vi "C-V 曲线测试.vi"() -> ()   [LabVIEW 2011]
panel:
  out "XY图":cluster{dbl[], dbl[]}[](graph)
  in  "测试时间（h）":dbl=0.5
  in  "低温循环测试":bool
  in  "延时（ms）":u32=100
  in  "步进电压(V)":dbl=2.0
  in  "最小电压(V)":dbl
  in  "最大电压(V)":dbl=30.0
  out "error out":errorcluster caption="错误输出"
  in  "Completion Task":u16(ring) caption="完成任务" items=["保持Excel打开", "关闭电子表格"]
  out "错误输出 2":errorcluster caption="错误输出"
  out "错误输出":errorcluster
  in  "Filename":string="TEST"
  in  "第n次记录":dbl
  in  "UNIT":string(combo)="1000000000000"
  in  "错误输入（无错误）":errorcluster
  in  "VISA资源名称":refnum<visa-resource-name>="GPIB0::1::INSTR"
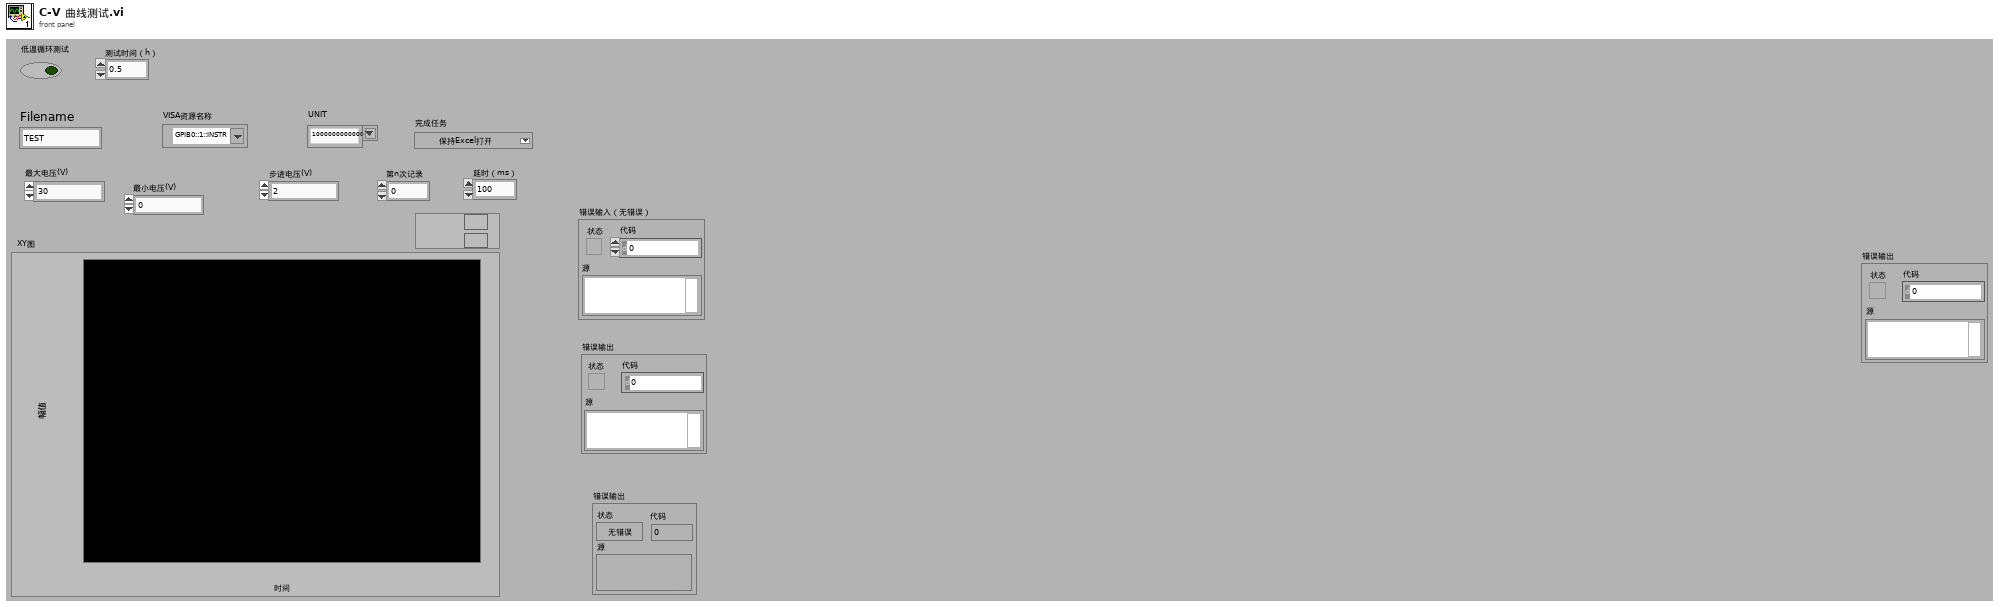
[diagram p1: front panel]
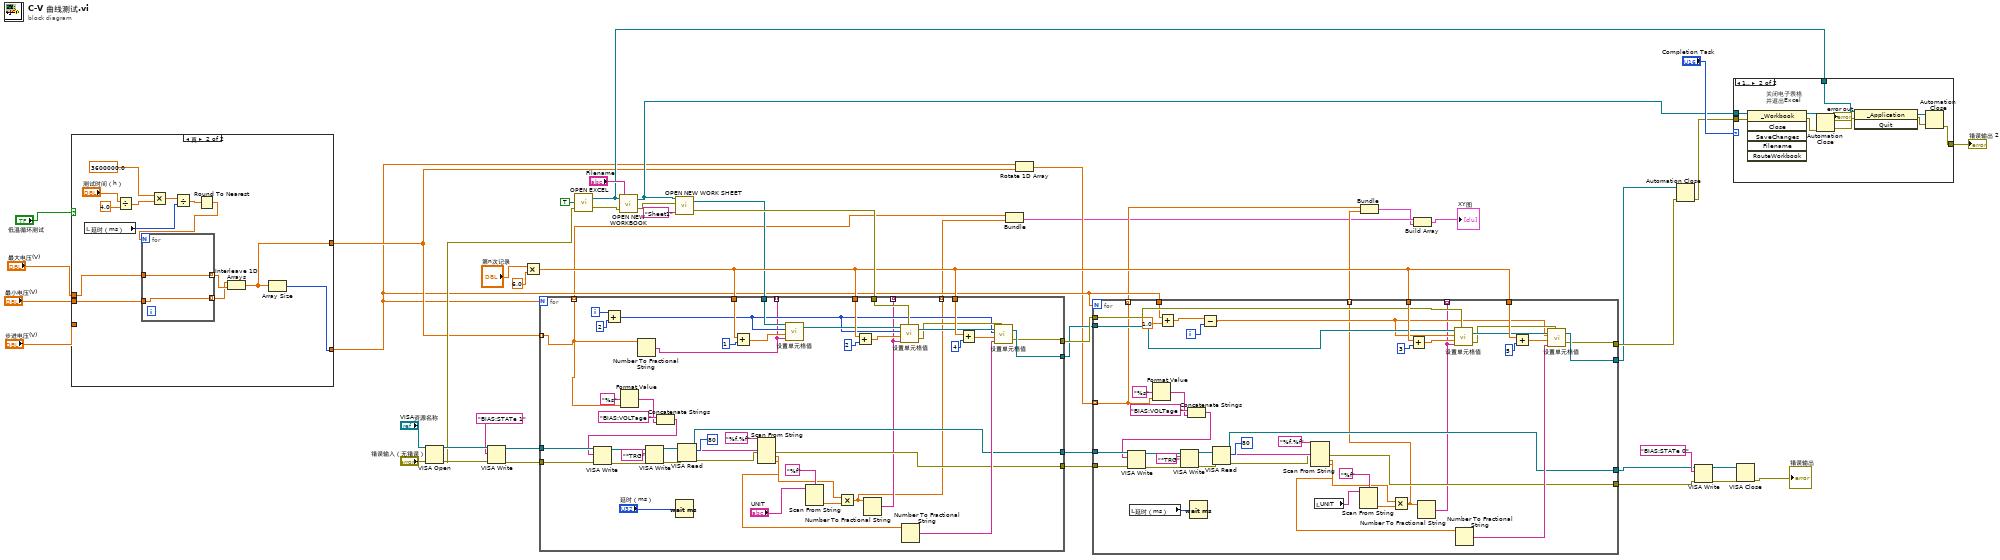
[diagram p0: block diagram]
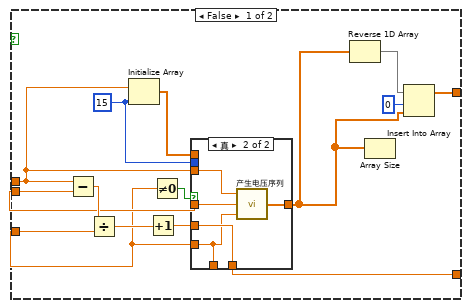
[diagram p2: hidden frame]
diagram:
  n1 = case shown="真" "低温循环测试" {
    tunnel: "最小电压(V)" -> [w53 w83]
    tunnel: "步进电压(V)" -> [w52 _]
    tunnel: "最大电压(V)" -> [w51 w84]
    tunnel: [w50 w74] -> w11
    tunnel: [w49 w73] -> w10
    frame False {
      w56 = 15 ("维数大小")
      n2 = Subtract(x=w51, y=w53) -> (x-y=w62:dbl)
      n3 = Divide(x=w62, y=w52) -> (x/y=w61:dbl)
      n4 = Initialize Array(w51, w56) -> (w57:dbl[])
      n5 = Increment(x=w61) -> (x+1=w58:dbl)
      n6 = Not Equal To 0?(x=w52) -> (x != 0?=w55:bool)
      n7 = case shown="真" w55 {
        tunnel: w53 -> [_ w70]
        tunnel: w51 -> [_ w69]
        tunnel: w52 -> [w63 w66]
        tunnel: [w65 w68] -> w54
        tunnel: w58 -> [_ w67]
        tunnel: [w64 w67] -> w49
        tunnel: w57 -> [w65 _]
        tunnel: w56 -> [w64 _]
        tunnel: [w63 w66] -> _
        frame False {
        }
        frame True {
          n8 = call "产生电压序列.vi"("Delt"=w66, "Min"=w70, "Max"=w69) -> ("Array"=w68:dbl[])
        }
      }
      n9 = Reverse 1D Array(array=w54) -> (reversed array=w59:dbl[])
      n10 = Array Size(array=w54) -> ()  [unwired: 1 out]
      n11 = Insert Into Array(array=w59, index=0 ("索引"), new element=w54) -> (w50:dbl[])
    }
    frame True {
      n12 = local read "延时（ms）"() -> (w77:u32)
      n13 = Divide(x="测试时间（h）", y=4.0) -> (x/y=w80:dbl)
      n14 = Multiply(x=3600000.0, y=w80) -> (x*y=w78:dbl)
      n15 = Divide(x=w78, y=w77) -> (x/y=w76:dbl)
      n16 = Round To Nearest(number=w76) -> (nearest integer value=w75:dbl)
      n17 = for {
        N: w75 -> [_]
        tunnel: w83 -> [w85]
        tunnel: w84 -> [w86]
        tunnel: [w86] -> w72 mode=indexing
        tunnel: [w85] -> w71 mode=indexing
      }
      n18 = Interleave 1D Arrays(w71, w72) -> (w74:dbl[])
      n19 = Array Size(array=w74) -> (size(s)=w73:i32)
    }
  }
  n20 = VISA Open(error in (no error)="错误输入（无错误）", VISA resource name="VISA资源名称") -> (VISA resource name=w47:refnum<visa-resource-name>, error out=w39:errorcluster)  [unwired: 3 in]
  n21 = VISA Write(VISA resource name=w47, write buffer="BIAS:STATe 1" ("写入缓冲区"), error in (no error)=w39) -> (VISA resource name out=w46:refnum<visa-resource-name>, error out=w45:errorcluster)  [unwired: 1 out]
  n22 = Multiply(x="第n次记录", y=6.0) -> (x*y=w22:dbl)
  n23 = call "OPEN EXCEL.vi"("错误输入（无错误）"=w39, "Visible"=TRUE) -> ("错误输出"=w38:errorcluster, "引用输出"=w30:refnum<k7>)  [unwired: 1 in]
  n24 = call "OPEN NEW WORKBOOK.vi"("错误输入（无错误）"=w38, "Filename"="Filename", "Excel._Application"=w30) -> ("错误输出"=w27:errorcluster, "Excel._Application 2"=w28:refnum<k7>)
  n25 = call "OPEN NEW WORK SHEET.vi"("Sheet?"="Sheet1", "错误输入（无错误）"=w27, "Excel._Workbook"=w28) -> ("错误输出"=w25:errorcluster, "Excel._Worksheet"=w21:refnum<k7>)  [unwired: 1 in]
  n26 = for {
    N: w10 -> [_]
    tunnel: w46 -> [w133]
    tunnel: w45 -> [w132]
    tunnel: w22 -> [w114]
    tunnel: w22 -> [w110]
    tunnel: [w100] -> w23
    tunnel: [w103] -> w16
    tunnel: [w102] -> w24
    tunnel: [w101] -> w17
    tunnel: w21 -> [w98]
    tunnel: w25 -> [w99]
    tunnel: w22 -> [w94]
    tunnel: w11 -> [w87] mode=indexing
    tunnel: [w90] -> _ mode=indexing
    tunnel: [w89] -> _ mode=indexing
    tunnel: [w88] -> w6 mode=indexing
    tunnel: [w87] -> w7 mode=indexing
    i -> [w108]
    n27 = Add(x=w108, y=2) -> (x+y=w93:i32)
    n28 = Format Value(format string="%s" ("格式字符串"), value (0)=w87) -> (output string=w124:string)  [unwired: 1 in]
    n29 = Number To Fractional String(number=w87) -> (F-format string=w90:string)  [unwired: 3 in]
    n30 = Concatenate Strings("BIAS:VOLTage " ("字符串"), w124) -> (w123:string)
    n31 = VISA Write(VISA resource name=w133, write buffer=w123, error in (no error)=w132) -> (VISA resource name out=w131:refnum<visa-resource-name>, error out=w130:errorcluster)  [unwired: 1 out]
    n32 = VISA Write(VISA resource name=w131, write buffer="*TRG" ("写入缓冲区"), error in (no error)=w130) -> (VISA resource name out=w129:refnum<visa-resource-name>, error out=w128:errorcluster)  [unwired: 1 out]
    n33 = Wait (ms)(milliseconds to wait="延时（ms）") -> ()  [unwired: 1 out]
    n34 = VISA Read(VISA resource name=w129, byte count=u32 80 ("字节总数"), error in (no error)=w128) -> (VISA resource name out=w102:refnum<visa-resource-name>, read buffer=w121:string, error out=w119:errorcluster)  [unwired: 1 out]
    n35 = Add(x=w94, y=1) -> (x+y=w95:dbl)
    n36 = Scan From String(format string="%f,%f" ("格式字符串"), input string=w121, error in=w119) -> (error out=w100:errorcluster, output 1=w116:dbl, output 2=w105:dbl)  [unwired: 3 in, 2 out]
    n37 = call "设置单元格值.vi"("Excel._Worksheet 2"=w98, "Row"=w93, "Col"=w95, "Value"=w90) -> ("Excel._Worksheet"=w97:refnum<k7>)  [unwired: 1 in, 1 out]
    n38 = Scan From String(format string="%f" ("格式字符串"), input string="UNIT") -> (output 1=w117:dbl)  [unwired: 3 in, 3 out]
    n39 = Multiply(x=w116, y=w117) -> (x*y=w88:dbl)
    n40 = Add(x=w114, y=2) -> (x+y=w113:dbl)
    n41 = Number To Fractional String(number=w88) -> (F-format string=w89:string)  [unwired: 3 in]
    n42 = call "设置单元格值.vi"("Excel._Worksheet 2"=w97, "Row"=w93, "Col"=w113, "Value"=w89, "error in (no error)"=w99) -> ("Excel._Worksheet"=w107:refnum<k7>, "error out"=w106:errorcluster)
    n43 = Number To Fractional String(number=w105) -> (F-format string=w104:string)  [unwired: 3 in]
    n44 = Add(x=w110, y=4) -> (x+y=w112:dbl)
    n45 = call "设置单元格值.vi"("Excel._Worksheet 2"=w107, "Row"=w93, "Col"=w112, "Value"=w104, "error in (no error)"=w106) -> ("Excel._Worksheet"=w103:refnum<k7>, "error out"=w101:errorcluster)
  }
  n46 = Bundle(w7, w6) -> (w3:cluster{dbl[], dbl[]})  [unwired: 1 in]
  n47 = Rotate 1D Array(1:w11, 2:w10) -> (0:w9:dbl[])
  n48 = for {
    N: w10 -> [_]
    tunnel: w24 -> [w177]
    tunnel: w23 -> [w176]
    tunnel: w22 -> [w158]
    tunnel: w22 -> [w154]
    tunnel: [w146] -> w19
    tunnel: [w149] -> w15
    tunnel: [w148] -> w20
    tunnel: [w147] -> w18
    tunnel: w17 -> [w145]
    tunnel: w16 -> [w144]
    tunnel: w10 -> [w140]
    tunnel: [w136] -> _ mode=indexing
    tunnel: w9 -> [w135] mode=indexing
    tunnel: [w135] -> w5 mode=indexing
    tunnel: [w134] -> w4 mode=indexing
    i -> [w141]
    n49 = local read "延时（ms）"() -> (w137:u32)
    n50 = Format Value(format string="%s" ("格式字符串"), value (0)=w135) -> (output string=w168:string)  [unwired: 1 in]
    n51 = Add(x=w140, y=1.0) -> (x+y=w142:dbl)
    n52 = Concatenate Strings("BIAS:VOLTage " ("字符串"), w168) -> (w167:string)
    n53 = VISA Write(VISA resource name=w177, write buffer=w167, error in (no error)=w176) -> (VISA resource name out=w175:refnum<visa-resource-name>, error out=w174:errorcluster)  [unwired: 1 out]
    n54 = VISA Write(VISA resource name=w175, write buffer="*TRG" ("写入缓冲区"), error in (no error)=w174) -> (VISA resource name out=w173:refnum<visa-resource-name>, error out=w172:errorcluster)  [unwired: 1 out]
    n55 = Wait (ms)(milliseconds to wait=w137) -> ()  [unwired: 1 out]
    n56 = Subtract(x=w142, y=w141) -> (x-y=w138:dbl)
    n57 = VISA Read(VISA resource name=w173, byte count=u32 80 ("字节总数"), error in (no error)=w172) -> (VISA resource name out=w148:refnum<visa-resource-name>, read buffer=w165:string, error out=w163:errorcluster)  [unwired: 1 out]
    n58 = Scan From String(format string="%f,%f" ("格式字符串"), input string=w165, error in=w163) -> (error out=w146:errorcluster, output 1=w160:dbl, output 2=w151:dbl)  [unwired: 3 in, 2 out]
    n59 = local read "UNIT"() -> (w143:string)
    n60 = Scan From String(format string="%f" ("格式字符串"), input string=w143) -> (output 1=w161:dbl)  [unwired: 3 in, 3 out]
    n61 = Multiply(x=w160, y=w161) -> (x*y=w134:dbl)
    n62 = Add(x=w158, y=3) -> (x+y=w157:dbl)
    n63 = Number To Fractional String(number=w134) -> (F-format string=w136:string)  [unwired: 3 in]
    n64 = call "设置单元格值.vi"("Excel._Worksheet 2"=w144, "Row"=w138, "Col"=w157, "Value"=w136, "error in (no error)"=w145) -> ("Excel._Worksheet"=w153:refnum<k7>, "error out"=w152:errorcluster)
    n65 = Number To Fractional String(number=w151) -> (F-format string=w150:string)  [unwired: 3 in]
    n66 = Add(x=w154, y=5) -> (x+y=w156:dbl)
    n67 = call "设置单元格值.vi"("Excel._Worksheet 2"=w153, "Row"=w138, "Col"=w156, "Value"=w150, "error in (no error)"=w152) -> ("Excel._Worksheet"=w149:refnum<k7>, "error out"=w147:errorcluster)
  }
  n68 = Bundle(w5, w4) -> (w2:cluster{dbl[], dbl[]})  [unwired: 1 in]
  n69 = Build Array(w3, w2) -> (→"XY图":cluster{dbl[], dbl[]}[])
  n70 = Automation Close(3:w18, 5:w15) -> (0:w31:errorcluster)
  n71 = VISA Write(VISA resource name=w20, write buffer="BIAS:STATe 0" ("写入缓冲区"), error in (no error)=w19) -> (VISA resource name out=w34:refnum<visa-resource-name>, error out=w35:errorcluster)  [unwired: 1 out]
  n72 = case shown="1.." "Completion Task" {
    tunnel: w28 -> [_ w181]
    tunnel: w31 -> [_ w180]
    tunnel: w30 -> [_ w179]
    tunnel: [_ w178] -> w29
    frame ..0 {
    }
    frame 1.. {
      # "关闭电子表格\n并退出Excel"
      n73 = invoke class="_Workbook" method="Close"(reference=w181, error in=w180) -> (reference out=w186:refnum<k7>, error out=w185:errorcluster)  [unwired: 4 in, 4 out]
      n74 = Automation Close(3:w185, 5:w186) -> (0:w184:errorcluster)
      n75 = invoke class="_Application" method="Quit"(reference=w179, error in=w184) -> (reference out=w182:refnum<k7>, error out=w183:errorcluster)  [unwired: 1 in, 1 out]
      n76 = Automation Close(3:w183, 5:w182) -> (0:w178:errorcluster)
    }
  }
  "错误输出 2" <- w29
  n77 = VISA Close(VISA resource name=w34, error in (no error)=w35) -> (error out=→"错误输出":errorcluster)
